vi "CH3 ON (subVI).vi"() -> (3 "String":string)   [LabVIEW 2018]
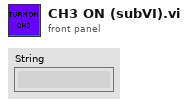
[diagram p1: front panel]
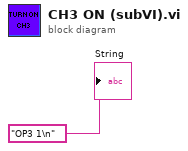
[diagram p0: block diagram]
diagram:
  "String" <- "OP3 1\n"
